vi "Load Config_Folder Filter.vi"(8 "error in (no error)":errorcluster, 11 "Refnum in":T2) -> (0 "error out":errorcluster, 2 "Folder Filter":T1, 3 "Refnum out":T2)   [LabVIEW 2019, in "AutoMenuCreator.lvlib"]
uses:
  AutoMenuCreator.lvlib
  <vilib>/Utility/config.llb/Config Data RefNum.ctl
  Ctl/Ctl_Config_Folder Filter.ctl
  <vilib>/Utility/config.llb/NI_LVConfig.lvlib
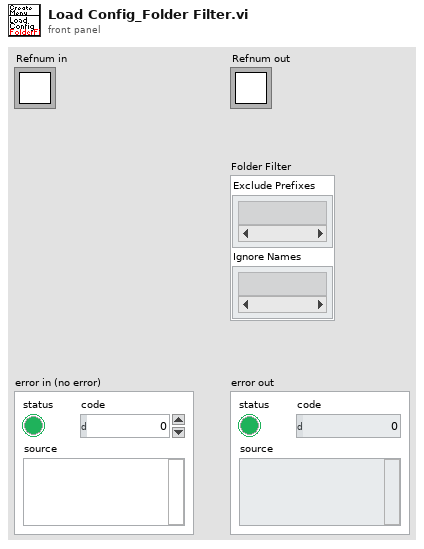
[diagram p1: front panel]
types:
  T1 = typedef "AutoMenuCreator.lvlib/Ctl_Config_Folder Filter.ctl" = cluster{"Exclude Prefixes":string[], "Ignore Names":string[]}
  T2 = typedef "NI_LVConfig.lvlib/Config Data RefNum.ctl" = refnum<k1>
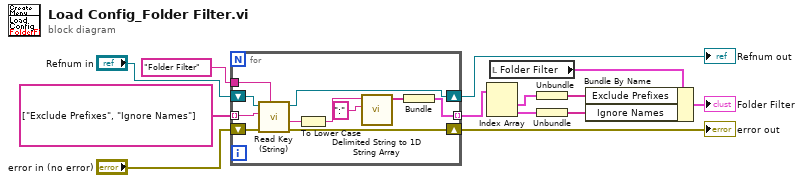
[diagram p0: block diagram]
diagram:
  n1 = for {
    tunnel: "Folder Filter" ("section") -> [w22]
    shift-right: [w21] -> w9
    shift-left: "Refnum in" -> [w23]
    shift-right: [w20] -> w8
    shift-left: "error in (no error)" -> [w24]
    tunnel: string[] ["Exclude Prefixes", "Ignore Names"] ("key") -> [w19] mode=indexing
    tunnel: [w15] -> w7 mode=indexing
    n2 = call <vilib>:"Read Key (String).vi"("section"=w22, "error in (no error)"=w24, "key"=w19, "refnum"=w23) -> ("error out"=w20:errorcluster, "value"=w18:string, "refnum out"=w21:T2)  [unwired: 4 in, 1 out]
    n3 = To Lower Case(string=w18) -> (all lower case string=w14:string)
    n4 = call <vilib>:"Delimited String to 1D String Array.vi"("delimiter"=":", "delimited string"=w14) -> ("string array"=w16:string[])  [unwired: 9 in]
    n5 = Bundle("string array"=w16) -> (w15:cluster{"string array":string[]})  [unwired: 1 in]
  }
  "error out" <- w8
  "Refnum out" <- w9
  n6 = Index Array(array=w7) -> (element #1=w6:cluster{"string array":string[]}, element #2=w5:cluster{"string array":string[]})  [unwired: 2 in]
  n7 = local read "Folder Filter"() -> (w1:T1)
  n8 = Unbundle(w6) -> ("string array"=w4:string[])
  n9 = Unbundle(w5) -> ("string array"=w3:string[])
  n10 = Bundle By Name(cluster=w1, "Exclude Prefixes"=w4, "Ignore Names"=w3) -> (→"Folder Filter":T1)
